vi "DT_Cal Length.vi"(10 "p 2":cluster{"x":dbl, "y":dbl, "index":i32}, 11 "p 1":cluster{"x":dbl, "y":dbl, "index":i32}) -> (3 "length":dbl)   [LabVIEW 2017, in "NI_AAL_Geometry.lvlib"]
uses:
  <vilib>/Analysis/NI_AAL_Geometry.lvlib
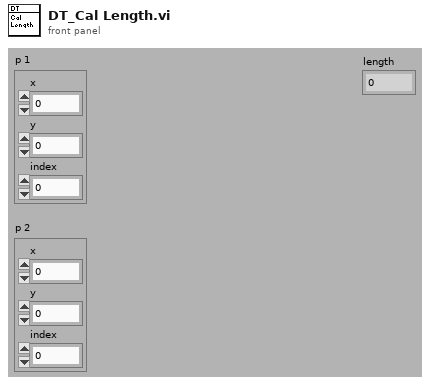
[diagram p1: front panel]
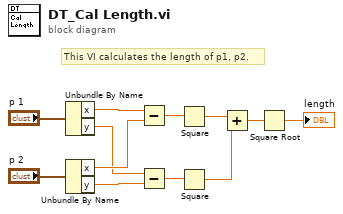
[diagram p0: block diagram]
diagram:
  # "This VI calculates the length of p1, p2."
  n1 = Unbundle By Name("p 1") -> ("x"=w10:dbl, "y"=w8:dbl)
  n2 = Unbundle By Name("p 2") -> ("x"=w9:dbl, "y"=w7:dbl)
  n3 = Subtract(x=w10, y=w9) -> (x-y=w6:dbl)
  n4 = Subtract(x=w8, y=w7) -> (x-y=w5:dbl)
  n5 = Square(x=w6) -> (x^2=w4:dbl)
  n6 = Square(x=w5) -> (x^2=w3:dbl)
  n7 = Add(x=w4, y=w3) -> (x+y=w2:dbl)
  n8 = Square Root(x=w2) -> (sqrt(x)=→"length":dbl)
